vi "Is an Error (error cluster)__JKI Error Handling.vi"(2 "error in":errorcluster) -> (7 "error?":bool)   [LabVIEW 2013]
doc: "Determines whether the <B>error in</B> error cluster contains an error (status = TRUE). If so, then the <B>error?</B> output will be TRUE.\n\n<B>This VI is polymorphic</B> -- it can also test arrays of error clusters. It has two possible modes of operation for handling arrays of errors:\n(1) <B>Error Cluster Array (any error?)</B>: outputs a single <B>any error?</B> Boolean which is TRUE if *any* element of <B>error array in</B> has an error.\n(2*) <B>Error Cluster Array</B>: outputs an array of <B>error?</B> Booleans that correspond to the elements of <B>error array in</B>.\n\n*Note, in order to select the <B>Error Cluster Array</B> mode, you must explicitly choose this option from the Polymorphic VI Selector ring or from the \"Select Type\" right-click submenu of the polymorphic VI."
panel:
  # "Copyright © 2006 James Kring, Inc. All rights reserved.\n\nAuthor: Jim Kring <jim.kring@jameskring.com>\n\nThis library is provided \"AS IS\" , WITHOUT WARRANTIES OR \nCONDITIONS OF ANY KIND, either express or implied.\n\nJames Kring, Inc. -- http://www.jameskring.com"
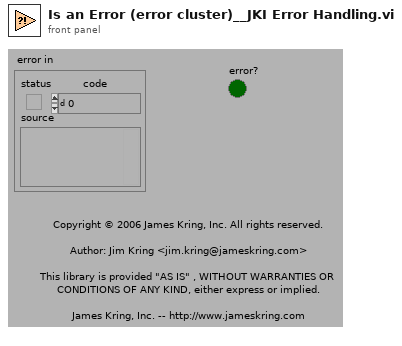
[diagram p1: front panel]
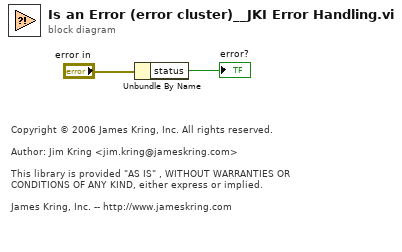
[diagram p0: block diagram]
diagram:
  # "Copyright © 2006 James Kring, Inc. All rights reserved.\n\nAuthor: Jim Kring <jim.kring@jameskring.com>\n\nThis library is provided \"AS IS\" , WITHOUT WARRANTIES OR \nCONDITIONS OF ANY KIND, either express or implied.\n\nJames Kring, Inc. -- http://www.jameskring.com"
  n1 = Unbundle By Name("error in") -> ("status"=→"error?":bool)
